vi "PID Internals_P.vi"(0 "Run PI?":bool, 1 "PIcluster":cluster{"SlewRate":dbl, "Kp":dbl, "Ki":dbl}, 2 "FFcluster":cluster{"FF_m":dbl, "FF_b":dbl}, 3 "LimitCluster":T1, 5 "SP":dbl, 7 "Error":dbl, 11 "RevCtrlZero":bool, 12 "NeedleValve":bool, 13 "Indirect FF":bool) -> (4 "PreSlew":dbl, 8 "Output":dbl)   [LabVIEW 2013]
uses:
  <vilib>/addons/control/pid/pid.llb/PID Output Rate Limiter (DBL).vi
  <vilib>/addons/control/pid/NI_PID_pid.lvlib
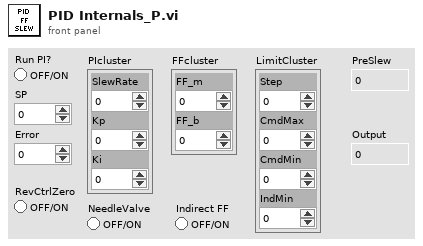
[diagram p1: front panel]
types:
  T1 = cluster{"Step":dbl, "CmdMax":dbl, "CmdMin":dbl, "IndMin":dbl}
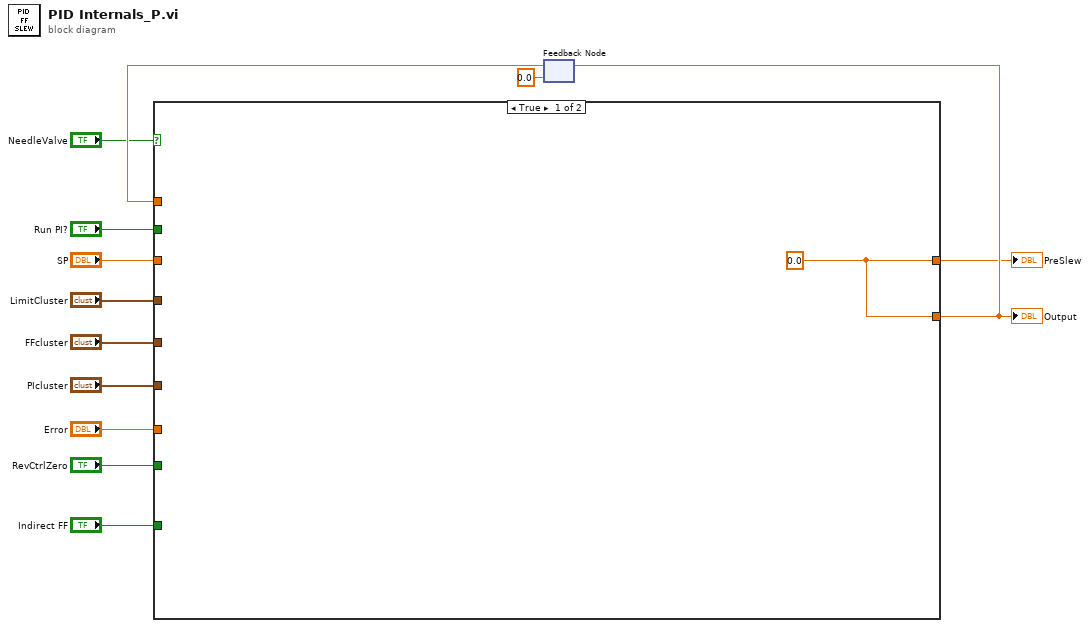
[diagram p0: block diagram]
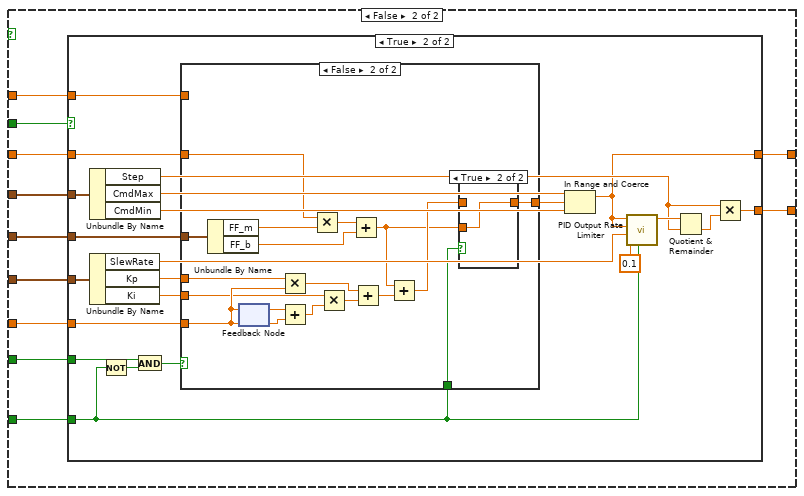
[diagram p2: hidden frame]
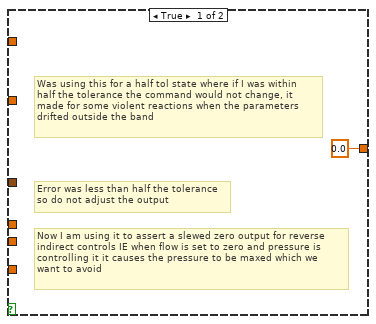
[diagram p4: hidden frame]
diagram:
  n1 = feedback #1(0.0 ("SP")) -> (w5:dbl)
  n2 = case shown="True" "NeedleValve" {
    tunnel: "Run PI?" -> [_ w25]
    tunnel: "SP" -> [_ w24]
    tunnel: "Error" -> [_ w23]
    tunnel: "FFcluster" -> [_ w22]
    tunnel: "PIcluster" -> [_ w21]
    tunnel: "LimitCluster" -> [_ w20]
    tunnel: "RevCtrlZero" -> [_ w19]
    tunnel: [w14 w18] -> w6
    tunnel: w5 -> [_ w17]
    tunnel: [w14 w16] -> w3
    tunnel: "Indirect FF" -> [_ w15]
    frame True {
      w14 = 0.0 ("CmdMax")
    }
    frame False {
      n3 = case shown="True" w25 {
        tunnel: [w26 w36] -> w18
        tunnel: w24 -> [w26 w48]
        tunnel: w23 -> [_ w47]
        tunnel: w22 -> [_ w46]
        tunnel: w21 -> [_ w43]
        tunnel: w20 -> [_ w44]
        tunnel: w19 -> [_ w29]
        tunnel: w17 -> [_ w45]
        tunnel: [w26 w31] -> w16
        tunnel: w15 -> [_ w27]
        frame False {
        }
        frame True {
          n4 = Unbundle By Name(w44) -> ("Step"=w37:dbl, "CmdMax"=w34:dbl, "CmdMin"=w33:dbl)
          n5 = Unbundle By Name(w43) -> ("SlewRate"=w38:dbl, "Kp"=w42:dbl, "Ki"=w41:dbl)
          n6 = Not(x=w27) -> (.not. x?=w30:bool)
          n7 = And(x=w29, y=w30) -> (x .and. y?=w28:bool)
          n8 = case shown="False" w28 {
            tunnel: w48 -> [_ w64]
            tunnel: w47 -> [_ w62]
            tunnel: w46 -> [_ w58]
            tunnel: w45 -> [_ _]
            tunnel: w42 -> [_ w55]
            tunnel: w41 -> [_ w54]
            tunnel: [0.0 ("CmdMax") w52] -> w35
            tunnel: w27 -> [_ w50]
            frame True {
              # "Now I am using it to assert a slewed zero output for reverse\nindirect controls IE when flow is set to zero and pressure is\ncontrolling it it causes the pressure to be maxed which we\nwant to avoid"
              # "Was using this for a half tol state where if I was within\nhalf the tolerance the command would not change, it\nmade for some violent reactions when the parameters\ndrifted outside the band"
              # "Error was less than half the tolerance\nso do not adjust the output"
            }
            frame False {
              n9 = Unbundle By Name(w58) -> ("FF_m"=w57:dbl, "FF_b"=w56:dbl)
              n10 = feedback #2(w62) -> (w63:dbl)
              n11 = feedback-in #2(w62) -> ()
              n12 = Multiply(x=w55, y=w62) -> (x*y=w60:dbl)
              n13 = Add(x=w63, y=w62) -> (x+y=w59:dbl)
              n14 = Multiply(x=w64, y=w57) -> (x*y=w66:dbl)
              n15 = Multiply(x=w54, y=w59) -> (x*y=w61:dbl)
              n16 = Add(x=w66, y=w56) -> (x+y=w51:dbl)
              n17 = Add(x=w60, y=w61) -> (x+y=w65:dbl)
              n18 = Add(x=w51, y=w65) -> (x+y=w53:dbl)
              n19 = case shown="True" w50 {
                tunnel: w53 -> [w67 _]
                tunnel: [w67 w68] -> w52
                tunnel: w51 -> [_ w68]
                frame False {
                }
                frame True {
                }
              }
            }
          }
          n20 = In Range and Coerce(upper limit=w34, x=w35, lower limit=w33) -> (coerced(x)=w31:dbl)  [unwired: 1 out]
          n21 = call-poly <vilib>:"PID Output Rate Limiter.vi"("reinitialize? (F)"=w27, "dt (s)"=0.1, "output rate (EGU/min)"=w38, "initial output"=w31, "input (controller output)"=w31) -> ("output"=w40:dbl)  [unwired: 3 in, 1 out]
          n22 = Quotient & Remainder(x=w40, y=w37) -> (floor(x/y)=w39:dbl)  [unwired: 1 out]
          n23 = Multiply(x=w37, y=w39) -> (x*y=w36:dbl)
        }
      }
    }
  }
  "Output" <- w6
  "PreSlew" <- w3
  n24 = feedback-in #1(w6) -> ()
